vi "Stop Acquisition.vi"(8 "error in (no error)":errorcluster, 10 "task in":refnum<k21>, 11 "Hardware Resources in":T1) -> (0 "error out":errorcluster)   [LabVIEW 2026, in "Acquisition.lvlib"]
doc: "Stops the acquisition."
uses:
  Acquisition.lvlib
  Instrument Specifications Configuration.ctl
  Instrument Specifications Cluster Configuration.ctl
  controls/UI/Measurement Role.ctl
  Settings/Settings.lvlib
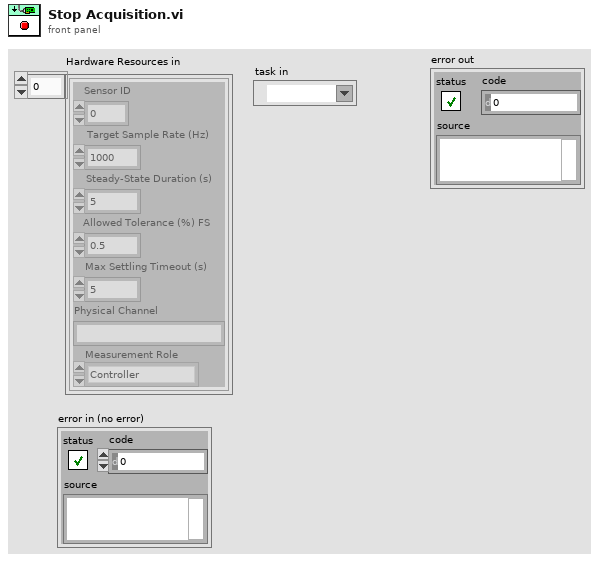
[diagram p1: front panel]
types:
  T1 = typedef "Acquisition.lvlib/Instrument Specifications Configuration.ctl" = T2[]
  T2 = typedef "Acquisition.lvlib/Instrument Specifications Cluster Configuration.ctl" = cluster{"Sensor ID":i32, "Target Sample Rate (Hz)":dbl, "Steady-State Duration (s)":i32, "Allowed Tolerance (%) FS":dbl, "Max Settling Timeout (s)":i32, "Physical Channel":string, "Measurement Role":T3}
  T3 = typedef "Settings.lvlib/Measurement Role.ctl" = enum16{"Controller", "Reference", "UUT", "Disable", "All"}
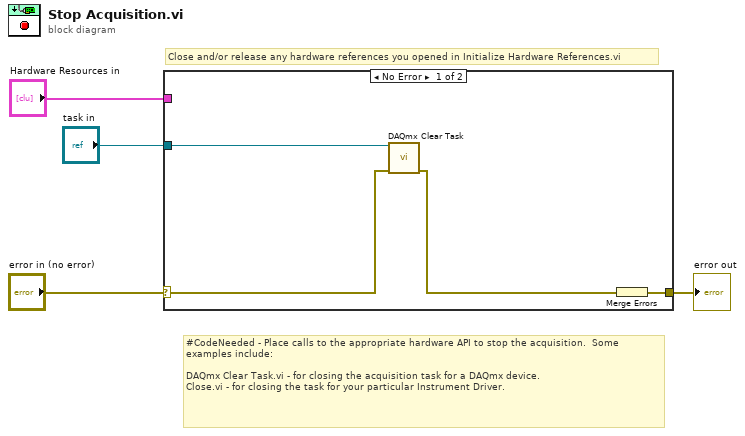
[diagram p0: block diagram]
diagram:
  # "#CodeNeeded - Place calls to the appropriate hardware API to stop the acquisition.  Some examples include:\n\nDAQmx Clear Task.vi - for closing the acquisition task for a DAQmx device.\nClose.vi - for closing the task for your particular Instrument Driver."
  # "Close and/or release any hardware references you opened in Initialize Hardware References.vi"
  n1 = case shown="No Error" "error in (no error)" {
    selector: "error in (no error)" -> [w7 w9]
    tunnel: [w8 w9] -> w3
    tunnel: "Hardware Resources in" -> [_ _]
    tunnel: "task in" -> [w5 _]
    frame No Error {
      n2 = call <vilib>:"DAQmx Clear Task.vi"("task in"=w5, "error in"=w7) -> ("error out"=w6:errorcluster)  [unwired: 13 in]
      n3 = Merge Errors(w6) -> (w8:errorcluster)
    }
    frame Error {
    }
  }
  "error out" <- w3
